vi "SUBVI_blackfly_format_info.vi"(1 "Cluster":T1) -> (0 "String":string)   [LabVIEW 2020]
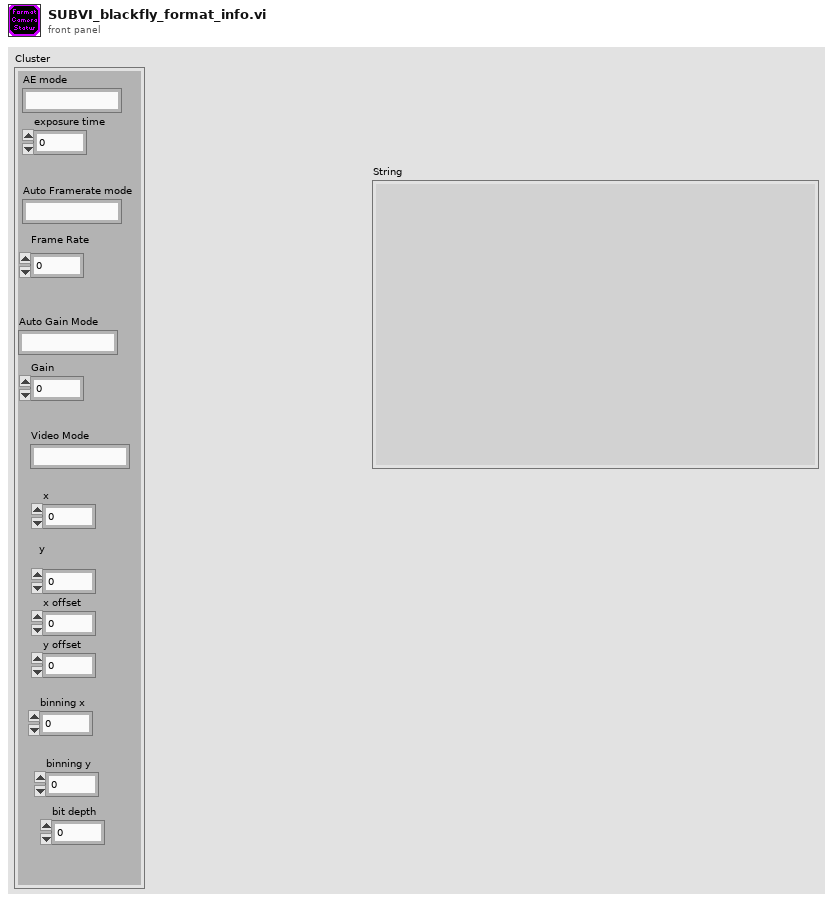
[diagram p1: front panel]
types:
  T1 = cluster{"AE mode":string, "exposure time":dbl, "Auto Framerate mode":string, "Frame Rate":dbl, "Auto Gain Mode":string, "Gain":dbl, "Video Mode":string, "x":dbl, "y":dbl, "x offset":dbl, "y offset":dbl, "binning x":dbl, "binning y":dbl, "bit depth":dbl}
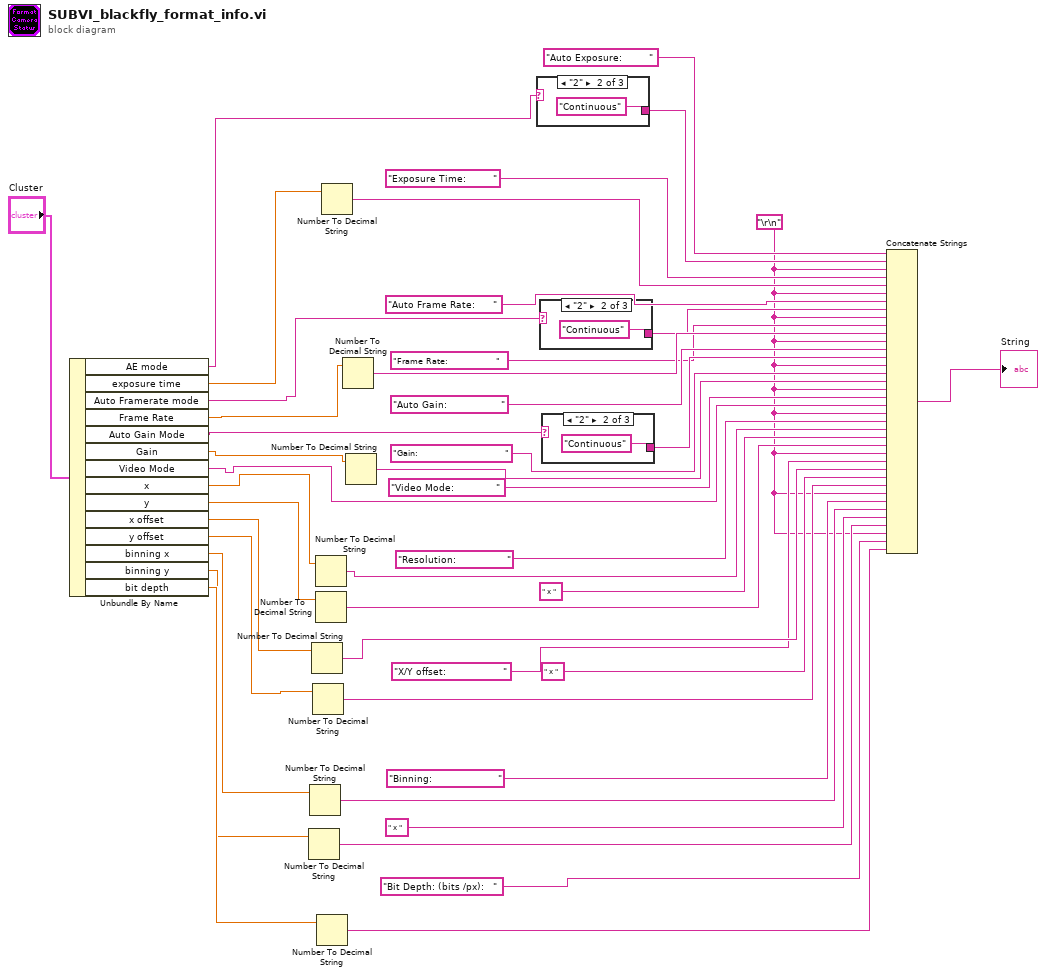
[diagram p0: block diagram]
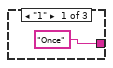
[diagram p2: hidden frame]
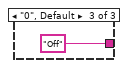
[diagram p3: hidden frame]
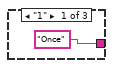
[diagram p4: hidden frame]
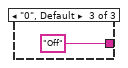
[diagram p5: hidden frame]
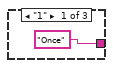
[diagram p6: hidden frame]
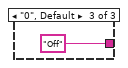
[diagram p7: hidden frame]
diagram:
  w3 = "\r\n"
  n1 = Unbundle By Name("Cluster") -> ("AE mode"=w16:string, "exposure time"=w15:dbl, "Auto Framerate mode"=w17:string, "Frame Rate"=w18:dbl, "Auto Gain Mode"=w14:string, "Gain"=w13:dbl, "Video Mode"=w12:string, "x"=w11:dbl, "y"=w10:dbl, "x offset"=w9:dbl, "y offset"=w8:dbl, "binning x"=w5:dbl, "binning y"=w6:dbl, "bit depth"=w7:dbl)
  n2 = Number To Decimal String(number=w6) -> (decimal integer string=w19:string)  [unwired: 1 in]
  n3 = Number To Decimal String(number=w5) -> (decimal integer string=w21:string)  [unwired: 1 in]
  n4 = Number To Decimal String(number=w9) -> (decimal integer string=w37:string)  [unwired: 1 in]
  n5 = Number To Decimal String(number=w8) -> (decimal integer string=w39:string)  [unwired: 1 in]
  n6 = Number To Decimal String(number=w11) -> (decimal integer string=w33:string)  [unwired: 1 in]
  n7 = Number To Decimal String(number=w10) -> (decimal integer string=w35:string)  [unwired: 1 in]
  n8 = Number To Decimal String(number=w7) -> (decimal integer string=w1:string)  [unwired: 1 in]
  n9 = Number To Decimal String(number=w15) -> (decimal integer string=w26:string)  [unwired: 1 in]
  n10 = Number To Decimal String(number=w18) -> (decimal integer string=w30:string)  [unwired: 1 in]
  n11 = Number To Decimal String(number=w13) -> (decimal integer string=w43:string)  [unwired: 1 in]
  n12 = case shown="\"2\"" w16 {
    tunnel: ["Once" "Continuous" "Off"] -> w24
    frame "1" {
    }
    frame "2" {
    }
    frame "0", Default {
    }
  }
  n13 = case shown="\"2\"" w17 {
    tunnel: ["Once" "Continuous" "Off"] -> w28
    frame "1" {
    }
    frame "2" {
    }
    frame "0", Default {
    }
  }
  n14 = case shown="\"2\"" w14 {
    tunnel: ["Once" "Continuous" "Off"] -> w32
    frame "1" {
    }
    frame "2" {
    }
    frame "0", Default {
    }
  }
  n15 = Concatenate Strings("Auto Exposure:         ", w24, w3, "Exposure Time:         ", w26, w3, "Auto Frame Rate:      ", w28, w3, "Frame Rate:                ", w30, w3, "Auto Gain:                  ", w32, w3, "Gain:                             ", w43, w3, "Video Mode:              ", w12, w3, "Resolution:                 ", w33, " x ", w35, w3, "X/Y offset:                   ", w37, " x ", w39, w3, "Binning:                      ", w21, " x ", w19, w3, "Bit Depth: (bits /px):   ", w1) -> (→"String":string)
